vi "Connect.vi"(9 "Location of FieldMax2Lib.dll in":path=path "C:/Windows/System32/FieldMax2Lib.dll") -> (1 "Meter Serial Number":string, 2 "Meter ID out":i32, 3 "Location of FieldMax2Lib.dll out":path)   [LabVIEW 2012]
panel:
  in  "Index":i16
  # "This VI needs to be run first to establish communication with the USB port on the FieldMaxII meter.  The Index value will typically be \"0\" if only one meter is connected.  When this VI is run, it will return a Meter ID value and a Meter Serial Number.  The Meter ID value should be wired through to each additional VI to tell the VI which meter to communicate with."
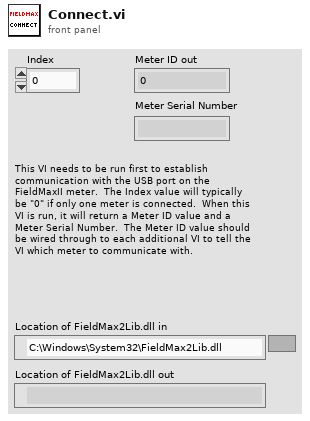
[diagram p1: front panel]
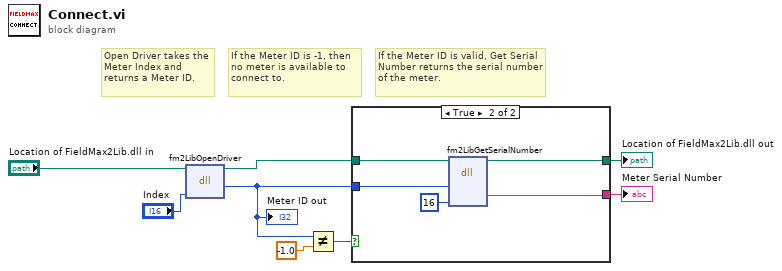
[diagram p0: block diagram]
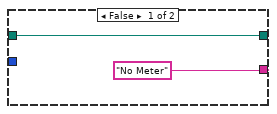
[diagram p2: hidden frame]
diagram:
  # "If the Meter ID is valid, Get Serial Number returns the serial number of the meter."
  # "If the Meter ID is -1, then no meter is available to connect to."
  # "Open Driver takes the Meter Index and returns a Meter ID."
  n1 = dll-call lib="C:/Windows/System32/FieldMax2Lib.dll" fn="fm2LibOpenDriver" label="Open Driver"(path in="Location of FieldMax2Lib.dll in", "index"="Index") -> (path out=w3:path, "return type"=w4:i32)  [unwired: 3 in, 1 out]
  "Meter ID out" <- w4
  n2 = Not Equal?(x=w4, y=-1.0) -> (x != y?=w7:bool)
  n3 = case shown="True" w7 {
    tunnel: w4 -> [_ w14]
    tunnel: ["No Meter" w13] -> w8
    tunnel: w3 -> [w9 w15]
    tunnel: [w9 w12] -> w5
    frame False {
    }
    frame True {
      n4 = dll-call lib="C:/Windows/System32/FieldMax2Lib.*" fn="fm2LibGetSerialNumber" label="Get Serial Number"(path in=w15, "h"=w14, "pSize"=i16 16) -> (path out=w12:path, "returnBuffer"=w13:string)  [unwired: 6 in, 1 out]
    }
  }
  "Meter Serial Number" <- w8
  "Location of FieldMax2Lib.dll out" <- w5
